vi "Modbus Master Example.vi"() -> ()   [LabVIEW 2017]
doc: "An example of the modbus master functionality."
uses:
  <vilib>/NI/Modbus Library/API/Master/Modbus Master.lvclass
  <vilib>/NI/Modbus Library/Master Function Definition/Read Device ID code.ctl
  <vilib>/NI/Modbus Library/API/Wrapper/Create Serial Master.vi
  <vilib>/NI/Modbus Library/API/Wrapper/API Main.lvlib
  <vilib>/NI/Modbus Library/Data Model/Device Data Model.lvclass
panel:
  in  "unit ID":u8=1
  in  "baud rate":u32=9600
  in  "VISA resource name":refnum<visa-resource-name>="COM14"
  in  "Stop Button":bool
  in  "Set Holding Registers":bool
  in  "Set Coils":bool
  in  "Fetch Discrete Inputs":bool
  in  "Fetch Input Registers":bool
  in  "Fetch Basic Objects":bool
  out "Basic Objects":string[](array[string])
  out "Status":string="Disconnected\nConnected\nInitializing\n"
  in  "Disconnect":bool
  in  "Connect":bool
  in  "Holding Registers":u16[](array[numeric])=[0, 0, 0, 0, 0, 0, 0, 0]
  out "Input Registers":u16[](array[numeric])=[5, 11, 0, 0, 0, 0, 0, 0]
  in  "Coils":bool[](array[boolean])=[TRUE, TRUE, TRUE, FALSE, FALSE, FALSE, FALSE, FALSE]
  out "Discrete Inputs":bool[](array[boolean])=[TRUE, TRUE, FALSE, FALSE, FALSE, FALSE, FALSE, FALSE]
  # "Coils are the boolean outputs of a modbus device. This example allows you to set the first 8 outputs."
  # "Holding Registers are the integer outputs of a modbus device. This example allows you to set the first 8 outputs."
  # "Modbus devices can also store objects in their memory, which are variable length strings. This example requests the basic level of objects."
  # "Discrete inputs are the boolean inputs of a modbus device. This example allows you to read the first 8 inputs."
  # "Input Registers are the integer inputs of a modbus device. This example allows you to read the first 8 inputs."
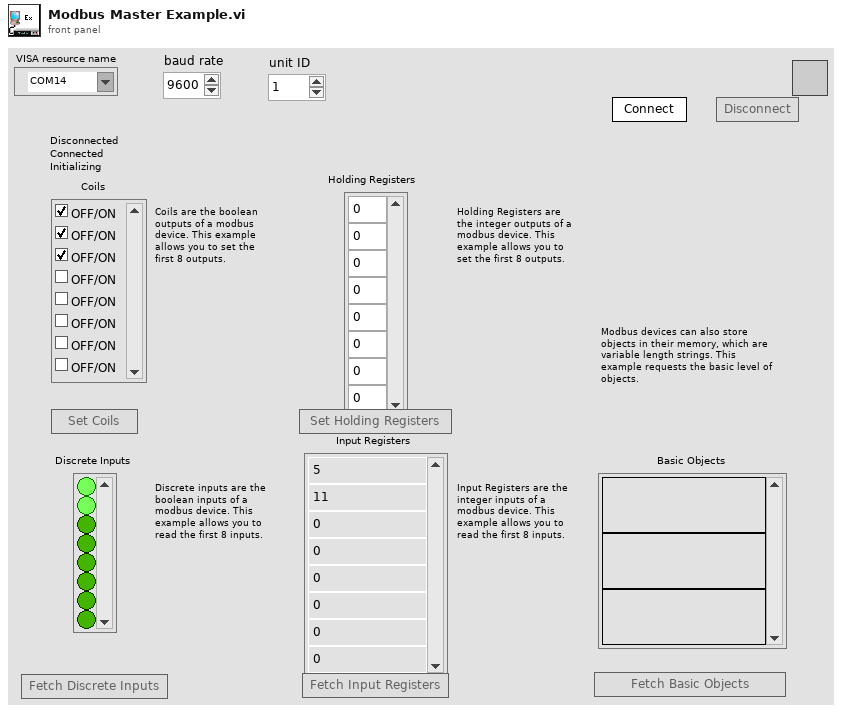
[diagram p1: front panel]
types:
  T1 = enum8{"Enabled", "Disabled", "Disabled and Grayed Out"}
  T2 = typedef "Device Data Model.lvclass/Read Device ID code.ctl" = enum8{"Read Basic", "Read Regular", "Read Extended", "Read Specific"}
  T3 = typedef "Device Data Model.lvclass/Identification Parameters.ctl" = cluster{"Object ID":u8, "Value":string}
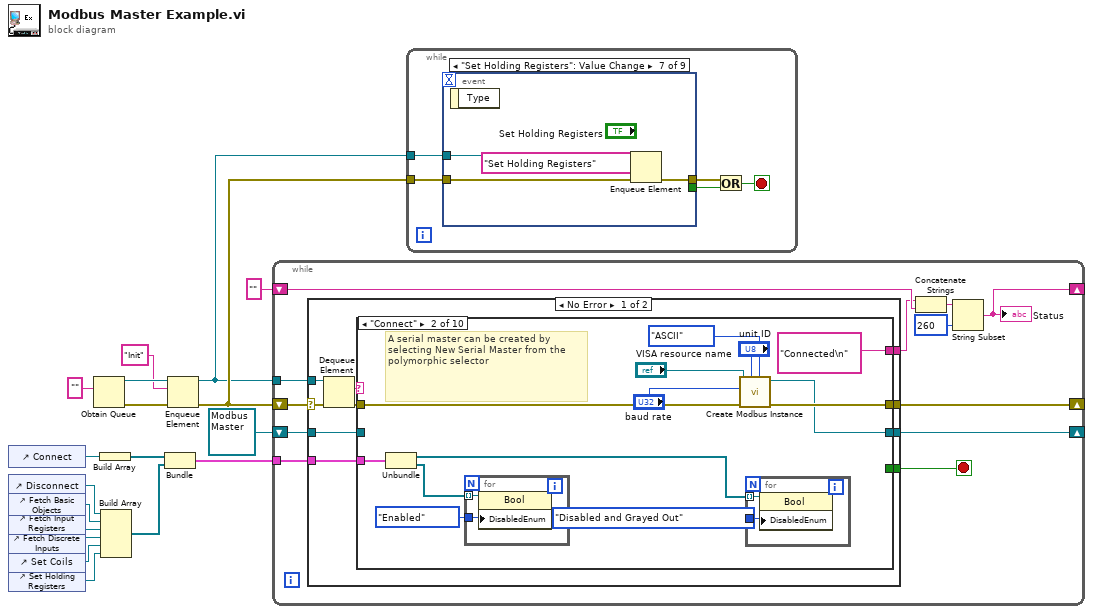
[diagram p0: block diagram]
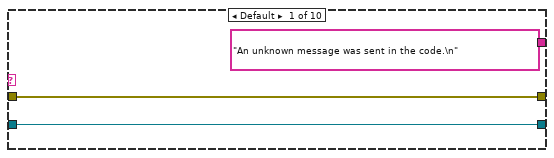
[diagram p2: hidden frame]
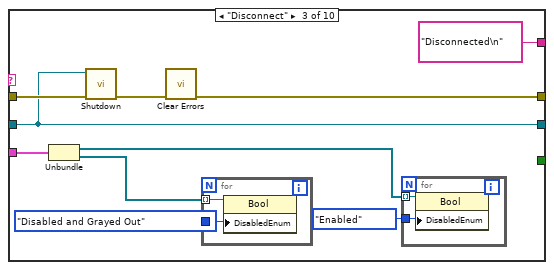
[diagram p3: hidden frame]
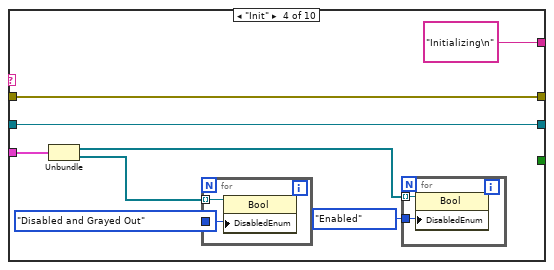
[diagram p4: hidden frame]
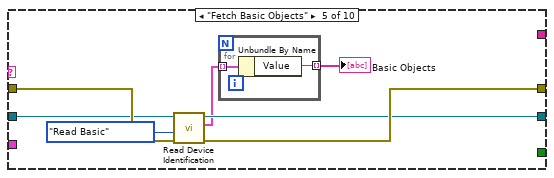
[diagram p5: hidden frame]
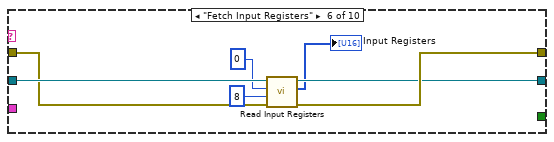
[diagram p6: hidden frame]
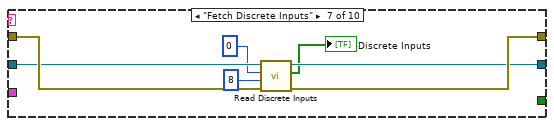
[diagram p7: hidden frame]
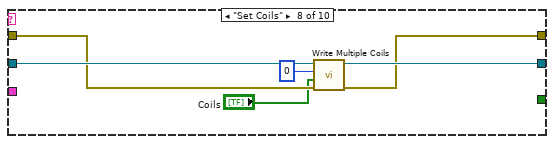
[diagram p8: hidden frame]
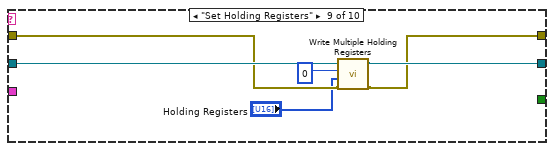
[diagram p9: hidden frame]
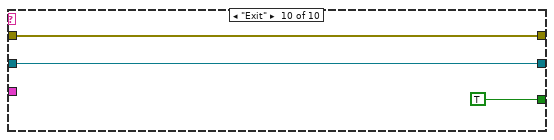
[diagram p10: hidden frame]
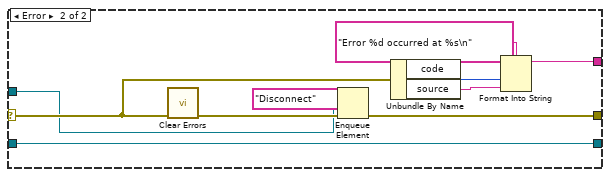
[diagram p11: hidden frame]
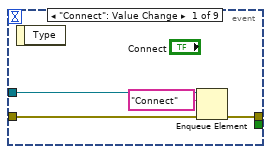
[diagram p12: hidden frame]
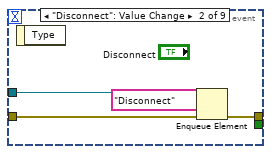
[diagram p13: hidden frame]
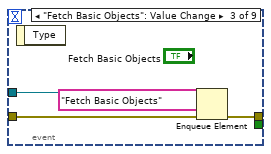
[diagram p14: hidden frame]
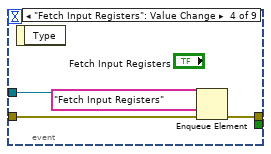
[diagram p15: hidden frame]
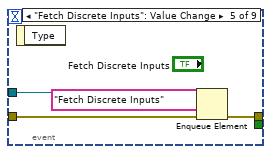
[diagram p16: hidden frame]
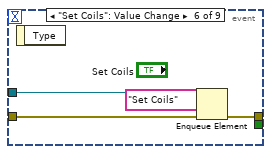
[diagram p17: hidden frame]
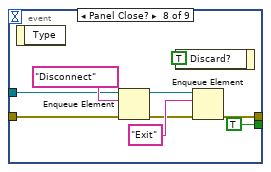
[diagram p18: hidden frame]
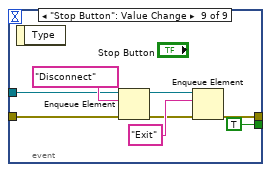
[diagram p19: hidden frame]
diagram:
  n1 = control-ref of="Connect"() -> (w9:refnum<vi>)
  n2 = control-ref of="Disconnect"() -> (w15:refnum<vi>)
  n3 = control-ref of="Fetch Basic Objects"() -> (w14:refnum<vi>)
  n4 = control-ref of="Fetch Input Registers"() -> (w13:refnum<vi>)
  n5 = control-ref of="Fetch Discrete Inputs"() -> (w12:refnum<vi>)
  n6 = control-ref of="Set Coils"() -> (w11:refnum<vi>)
  n7 = control-ref of="Set Holding Registers"() -> (w10:refnum<vi>)
  n8 = Obtain Queue(element data type="") -> (queue out=w4:refnum<queue>, error out=w18:errorcluster)  [unwired: 4 in, 1 out]
  n9 = Build Array(w9) -> (w6:refnum<vi>[])
  n10 = Build Array(w15, w14, w13, w12, w11, w10) -> (w8:refnum<vi>[])
  n11 = Bundle(w6, w8) -> (w7:cluster{refnum<vi>[], refnum<vi>[]})  [unwired: 1 in]
  n12 = Enqueue Element(queue=w4, element="Init", error in (no error)=w18) -> (queue out=w3:refnum<queue>, error out=w5:errorcluster)  [unwired: 1 in, 1 out]
  n13 = while {
    shift-right: [w22] -> _
    shift-left: refnum<class "Modbus Master.lvclass"> refnum ("Modbus Master") -> [w21]
    tunnel: w3 -> [w30]
    shift-right: [w28] -> _
    shift-left: w5 -> [w29]
    shift-right: [w27] -> _
    shift-left: "" ("Status") -> [w24]
    tunnel: w7 -> [w19]
    stop <- w20 stop-if-true
    n14 = case shown="No Error" w29 {
      selector: w29 -> [w39 w132]
      tunnel: w30 -> [w40 w126]
      tunnel: [w36 w133] -> w28
      tunnel: [w33 w129] -> w23
      tunnel: [w35 w125] -> w22
      tunnel: w21 -> [w34 w125]
      tunnel: [w32 _] -> w20
      tunnel: w19 -> [w31 _]
      frame No Error {
        n15 = Dequeue Element(queue=w40, error in (no error)=w39) -> (element=w37:string, error out=w38:errorcluster)  [unwired: 1 in, 2 out]
        n16 = case shown="\"Connect\"" w37 {
          tunnel: w38 -> [w43 w56 w70 w82 w93 w99 w109 w112 w118 w124]
          tunnel: [w43 w55 w66 w82 w92 w102 w108 w113 w119 w124] -> w36
          tunnel: [w42 w54 w68 w81 w90 w101 w106 w114 w120 w123] -> w35
          tunnel: w34 -> [w42 _ w68 w81 w91 w100 w107 w115 w121 w123]
          tunnel: ["An unknown message was sent in the code.\n" "Connected\n" "Disconnected\n" "Initializing\n" _ _ _ _ _ _] -> w33
          tunnel: [_ _ _ _ _ _ _ _ _ TRUE] -> w32
          tunnel: w31 -> [_ w52 w65 w79 _ _ _ _ _ _]
          frame Default {
          }
          frame "Connect" {
            # "A serial master can be created by selecting New Serial Master from the polymorphic selector"
            n17 = Unbundle(w52) -> (w50:refnum<vi>[], w51:refnum<vi>[])
            n18 = for {
              tunnel: w51 -> [w58] mode=indexing
              tunnel: T1."Enabled" ("Disabled") -> [w57]
              n19 = property class="Bool"(reference=w58, "DisabledEnum"=w57) -> ()  [unwired: 1 in, 2 out]
            }
            n20 = call-poly <vilib>:"Create Modbus Instance.vi"("serial type"=enum16{"RTU", "ASCII"}."ASCII", "unit ID"="unit ID", "error in"=w56, "baud rate"="baud rate", "VISA resource name"="VISA resource name") -> ("error out"=w55:errorcluster, "serial master instance"=w54:refnum<class "Modbus Master.lvclass">)  [unwired: 5 in]
            n21 = for {
              tunnel: w50 -> [w60] mode=indexing
              tunnel: T1."Disabled and Grayed Out" ("Disabled") -> [w59]
              n22 = property class="Bool"(reference=w60, "DisabledEnum"=w59) -> ()  [unwired: 1 in, 2 out]
            }
          }
          frame "Disconnect" {
            n23 = Unbundle(w65) -> (w63:refnum<vi>[], w64:refnum<vi>[])
            n24 = call-dynamic "Shutdown.vi"("error in"=w70, "Modbus master in"=w68) -> ("error out"=w69:errorcluster)  [unwired: 9 in]
            n25 = call <vilib>:"Clear Errors.vi"("error in (no error)"=w69) -> ("error out"=w66:errorcluster)  [unwired: 5 in, 1 out]
            n26 = for {
              tunnel: w64 -> [w74] mode=indexing
              tunnel: T1."Disabled and Grayed Out" ("Disabled") -> [w73]
              n27 = property class="Bool"(reference=w74, "DisabledEnum"=w73) -> ()  [unwired: 1 in, 2 out]
            }
            n28 = for {
              tunnel: w63 -> [w72] mode=indexing
              tunnel: T1."Enabled" ("Disabled") -> [w71]
              n29 = property class="Bool"(reference=w72, "DisabledEnum"=w71) -> ()  [unwired: 1 in, 2 out]
            }
          }
          frame "Init" {
            n30 = Unbundle(w79) -> (w77:refnum<vi>[], w78:refnum<vi>[])
            n31 = for {
              tunnel: w78 -> [w86] mode=indexing
              tunnel: T1."Disabled and Grayed Out" ("Disabled") -> [w85]
              n32 = property class="Bool"(reference=w86, "DisabledEnum"=w85) -> ()  [unwired: 1 in, 2 out]
            }
            n33 = for {
              tunnel: w77 -> [w84] mode=indexing
              tunnel: T1."Enabled" ("Disabled") -> [w83]
              n34 = property class="Bool"(reference=w84, "DisabledEnum"=w83) -> ()  [unwired: 1 in, 2 out]
            }
          }
          frame "Fetch Basic Objects" {
            n35 = call-dynamic "Read Device Identification.vi"("error in"=w93, "read device ID code"=Read_Device_ID_code."Read Basic" ("Read Device ID code"), "Modbus master in"=w91) -> ("error out"=w92:errorcluster, "objects"=w88:T3[], "Modbus master out"=w90:refnum<class "Modbus Master.lvclass">)  [unwired: 6 in]
            n36 = for {
              tunnel: w88 -> [w95] mode=indexing
              tunnel: [w94] -> w87 mode=indexing
              n37 = Unbundle By Name(w95) -> ("Value"=w94:string)
            }
            "Basic Objects" <- w87
          }
          frame "Fetch Input Registers" {
            n38 = call-dynamic "Read Input Registers.vi"("error in"=w99, "number of inputs"=u16 8 ("number of registers"), "starting address"=u16 0, "Modbus master in"=w100) -> ("error out"=w102:errorcluster, "register values"=→"Input Registers":u16[], "Modbus master out"=w101:refnum<class "Modbus Master.lvclass">)  [unwired: 5 in]
          }
          frame "Fetch Discrete Inputs" {
            n39 = call-dynamic "Read Discrete Inputs.vi"("error in"=w109, "number of inputs"=u16 8, "starting address"=u16 0, "Modbus master in"=w107) -> ("error out"=w108:errorcluster, "discrete inputs"=→"Discrete Inputs":bool[], "Modbus master out"=w106:refnum<class "Modbus Master.lvclass">)  [unwired: 5 in]
          }
          frame "Set Coils" {
            n40 = call-dynamic "Write Multiple Coils.vi"("error in"=w112, "coils to write"="Coils", "starting address"=u16 0, "Modbus master in"=w115) -> ("error out"=w113:errorcluster, "Modbus master out"=w114:refnum<class "Modbus Master.lvclass">)  [unwired: 6 in]
          }
          frame "Set Holding Registers" {
            n41 = call-dynamic "Write Multiple Holding Registers.vi"("error in"=w118, "registers to write"="Holding Registers", "starting address"=u16 0, "Modbus master in"=w121) -> ("error out"=w119:errorcluster, "Modbus master out"=w120:refnum<class "Modbus Master.lvclass">)  [unwired: 6 in]
          }
          frame "Exit" {
          }
        }
      }
      frame Error {
        n42 = call <vilib>:"Clear Errors.vi"("error in (no error)"=w132) -> ("error out"=w134:errorcluster)  [unwired: 5 in, 1 out]
        n43 = Enqueue Element(queue=w126, element="Disconnect", error in (no error)=w134) -> (error out=w133:errorcluster)  [unwired: 1 in, 2 out]
        n44 = Unbundle By Name(w132) -> ("code"=w131:i32, "source"=w130:string)
        n45 = Format Into String(format string="Error %d occurred at %s\n", w131, w130) -> (resulting string=w129:string)  [unwired: 2 in, 1 out]
      }
    }
    n46 = Concatenate Strings(w23, w24) -> (w25:string)
    n47 = String Subset(string=w25, length (rest)=260 ("length (rest)")) -> (substring=w27:string)  [unwired: 1 in]
    "Status" <- w27
  }
  n48 = while {
    tunnel: w5 -> [w139]
    tunnel: w3 -> [w138]
    stop <- w135 stop-if-true
    n49 = event shown="[6] \"Set Holding Registers\": Value Change" {
      selector: _ -> [_ _ _ _ _ _ _ _ _]
      dyn-events: _ -> [_ _ _ _ _ _ _ _ _]
      timeout: _ -> [_ _ _ _ _ _ _ _ _]
      tunnel: w139 -> [w143 w147 w151 w155 w159 w163 w167 w173 w182]
      tunnel: [w142 w146 w150 w154 w158 w162 w166 w168 w177] -> w137
      tunnel: w138 -> [w141 w145 w149 w153 w157 w161 w165 w170 w179]
      tunnel: [_ _ _ _ _ _ _ TRUE ("Discard?") TRUE ("Discard?")] -> w136
      event "Connect": Value Change {
        n50 = event-data() -> ()  [unwired: 1 in, 1 out]
        n51 = Enqueue Element(queue=w141, element="Connect", error in (no error)=w143) -> (error out=w142:errorcluster)  [unwired: 1 in, 2 out]
      }
      event "Disconnect": Value Change {
        n52 = event-data() -> ()  [unwired: 1 in, 1 out]
        n53 = Enqueue Element(queue=w145, element="Disconnect", error in (no error)=w147) -> (error out=w146:errorcluster)  [unwired: 1 in, 2 out]
      }
      event "Fetch Basic Objects": Value Change {
        n54 = event-data() -> ()  [unwired: 1 in, 1 out]
        n55 = Enqueue Element(queue=w149, element="Fetch Basic Objects", error in (no error)=w151) -> (error out=w150:errorcluster)  [unwired: 1 in, 2 out]
      }
      event "Fetch Input Registers": Value Change {
        n56 = event-data() -> ()  [unwired: 1 in, 1 out]
        n57 = Enqueue Element(queue=w153, element="Fetch Input Registers", error in (no error)=w155) -> (error out=w154:errorcluster)  [unwired: 1 in, 2 out]
      }
      event "Fetch Discrete Inputs": Value Change {
        n58 = event-data() -> ()  [unwired: 1 in, 1 out]
        n59 = Enqueue Element(queue=w157, element="Fetch Discrete Inputs", error in (no error)=w159) -> (error out=w158:errorcluster)  [unwired: 1 in, 2 out]
      }
      event "Set Coils": Value Change {
        n60 = event-data() -> ()  [unwired: 1 in, 1 out]
        n61 = Enqueue Element(queue=w161, element="Set Coils", error in (no error)=w163) -> (error out=w162:errorcluster)  [unwired: 1 in, 2 out]
      }
      event "Set Holding Registers": Value Change {
        n62 = event-data() -> ()  [unwired: 1 in, 1 out]
        n63 = Enqueue Element(queue=w165, element="Set Holding Registers", error in (no error)=w167) -> (error out=w166:errorcluster)  [unwired: 1 in, 2 out]
      }
      event Panel Close? {
        n64 = event-data() -> ()  [unwired: 1 in, 1 out]
        n65 = Enqueue Element(queue=w170, element="Disconnect", error in (no error)=w173) -> (queue out=w171:refnum<queue>, error out=w169:errorcluster)  [unwired: 1 in, 1 out]
        n66 = event-data("Discard?"=TRUE) -> ()  [unwired: 1 in, 1 out]
        n67 = Enqueue Element(queue=w171, element="Exit", error in (no error)=w169) -> (error out=w168:errorcluster)  [unwired: 1 in, 2 out]
      }
      event "Stop Button": Value Change {
        n68 = event-data() -> ()  [unwired: 1 in, 1 out]
        n69 = Enqueue Element(queue=w179, element="Disconnect", error in (no error)=w182) -> (queue out=w180:refnum<queue>, error out=w178:errorcluster)  [unwired: 1 in, 1 out]
        n70 = Enqueue Element(queue=w180, element="Exit", error in (no error)=w178) -> (error out=w177:errorcluster)  [unwired: 1 in, 2 out]
      }
    }
    n71 = Or(x=w137, y=w136) -> (x .or. y?=w135:bool)
  }
